vi "ResizeImageInArray.vi"(8 "error in (no error)":errorcluster, 10 "Draw Area Width/Height":i32[](array[numeric]), 11 "Array in":refnum<vi>) -> (0 "error out":errorcluster)   [LabVIEW 2022 SP3]
uses:
  <vilib>/Utility/miscctls.llb/LVBoundsTypeDef.ctl
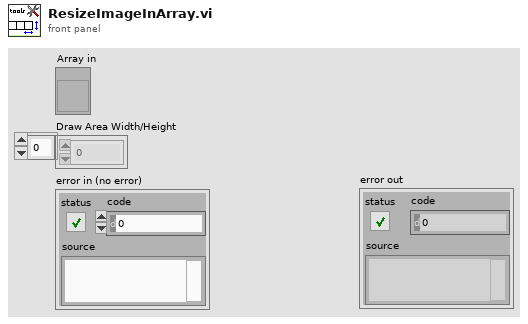
[diagram p1: front panel]
types:
  T1 = typedef "LVBoundsTypeDef.ctl" = cluster{"Width":i32, "Height":i32}
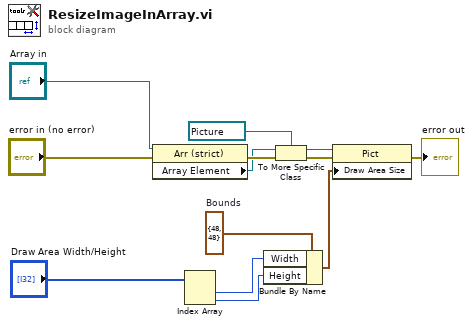
[diagram p0: block diagram]
diagram:
  w7 = T1 {"Width"=48, "Height"=48}  # Bounds
  n1 = property on="Property Node" class="Arr (strict)"(reference="Array in", error in="error in (no error)") -> (error out=w13:errorcluster, "Array Element"=w3:refnum<vi>)  [unwired: 1 out]
  n2 = Index Array(array="Draw Area Width/Height") -> (element #1=w5:i32, element #2=w6:i32)  [unwired: 2 in]
  n3 = Bundle By Name(cluster=w7, "Width"=w5, "Height"=w6) -> (w9:T1)
  n4 = To More Specific Class(target class=refnum<vi> refnum ("2D Picture 2"), reference=w3, error in=w13) -> (specific class reference=w4:refnum<vi>, error out=w12:errorcluster)
  n5 = property on="Property Node" class="Pict"(reference=w4, error in=w12, "Draw Area Size"=w9) -> (error out=→"error out":errorcluster)  [unwired: 1 out]
